vi "ClearObjectCache.vi"(5 "error in (no error)":errorcluster) -> (19 "error out":errorcluster)   [LabVIEW 2017, in "G#RemoteProxy.lvclass"]
doc: "Clears the object cache."
uses:
  G#RemoteProxy.lvclass
  G#Object/G#Object.lvclass
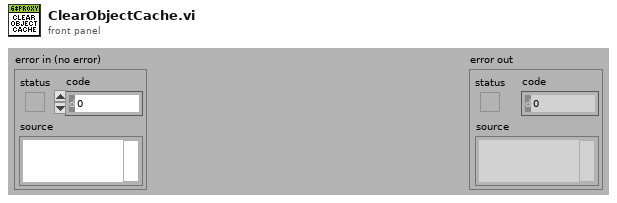
[diagram p1: front panel]
types:
  T1 = typedef "G#RemoteProxy.lvclass/ClassAttributesRef.ctl" = refnum<data-value>
  T2 = typedef "G#RemoteProxy.lvclass/ClassAttributesProxy.ctl" = cluster{"NoActiveProject":bool, "FullClassNames":string[], "FullClassPaths":path[], "RemoteRefs":refnum<class "G#Object.lvclass">[], "ProxyRefs":refnum<class "G#RemoteProxy.lvclass">[], "RemoteClassName":string[], "ProxyClassRefs":refnum<class "G#RemoteProxy.lvclass">[]}
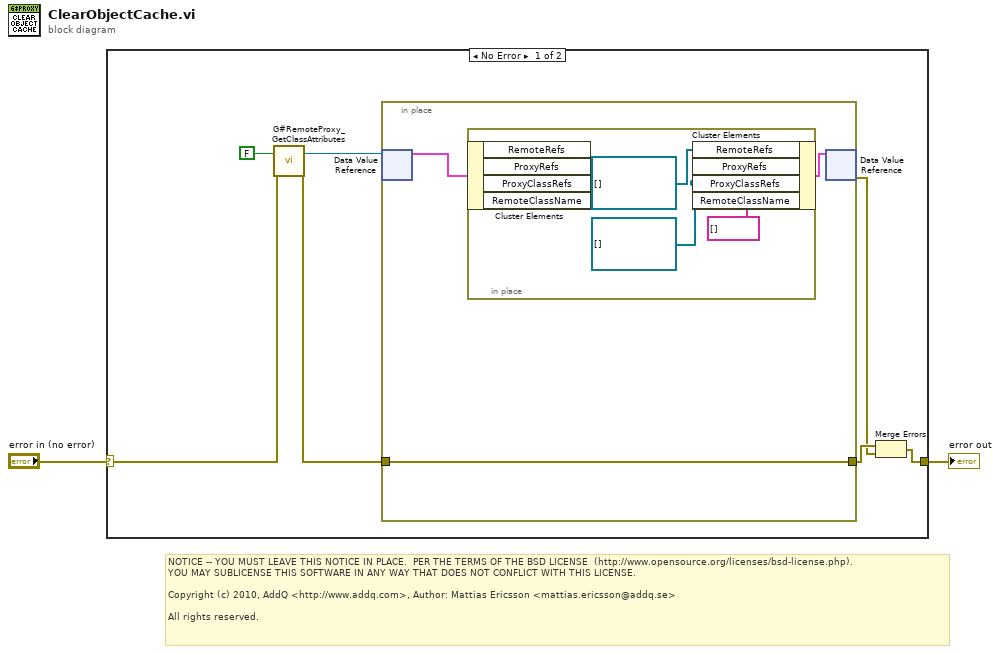
[diagram p0: block diagram]
diagram:
  # "NOTICE -- YOU MUST LEAVE THIS NOTICE IN PLACE.  PER THE TERMS OF THE BSD LICENSE  (http://www.opensource.org/licenses/bsd-license.php).\nYOU MAY SUBLICENSE THIS SOFTWARE IN ANY WAY THAT DOES NOT CONFLICT WITH THIS LICENSE.\n\nCopyright (c) 2010, AddQ <http://www.addq.com>, Author: Mattias Ericsson <mattias.ericsson@addq.se>\n\nAll rights reserved."
  n1 = case shown="No Error" "error in (no error)" {
    selector: "error in (no error)" -> [w9 w16]
    tunnel: [w6 w16] -> w1
    frame No Error {
      n2 = call "G#RemoteProxy_GetClassAttributes.vi"("return data? (T)"=FALSE ("return data"), "error in (no error)"=w9) -> ("class attributes ref"=w7:T1, "error out"=w8:errorcluster)  [unwired: 14 in, 2 out]
      n3 = in-place {
        in-place-border: w8 -> [w10]
        in-place-border: [w10] -> w4
        n4 = in-place-dvr #1(w7) -> (w11:T2)  [unwired: 1 out]
        n5 = in-place {
          w14 = refnum<class "G#RemoteProxy.lvclass">[] [] ("ProxyObjectRefs")
          n6 = in-place-cluster #2(w11) -> ()  [unwired: 4 out]
          n7 = in-place-cluster #2("RemoteRefs"=refnum<class "G#Object.lvclass">[] [] ("RemoteObjectRefs"), "ProxyRefs"=w14, "ProxyClassRefs"=w14, "RemoteClassName"=string[] []) -> (w12:T2)
        }
        n8 = in-place-dvr #1(w12) -> (w3:errorcluster)  [unwired: 1 out]
      }
      n9 = Merge Errors(w4, w3) -> (w6:errorcluster)
    }
    frame Error {
    }
  }
  "error out" <- w1
